vi "MTM2_issueCommand_setAuthList.vi"(8 "error in (no error)":errorcluster, 11 "command_setAuthList_Ctl":T1) -> (0 "error out":errorcluster, 2 "function return":i32, 3 "command_setAuthList_Ctl out":T1)   [LabVIEW 2018, in "SALLV_MTM2.lvlib"]
doc: "int MTM2_shm_issueCommand_setAuthListLV(MTM2_command_setAuthListLV *command_setAuthList_Ctl );"
uses:
  DataTypes/command_setAuthList.ctl
  SALLV_MTM2.lvlib
  SALLV_MTM2.so
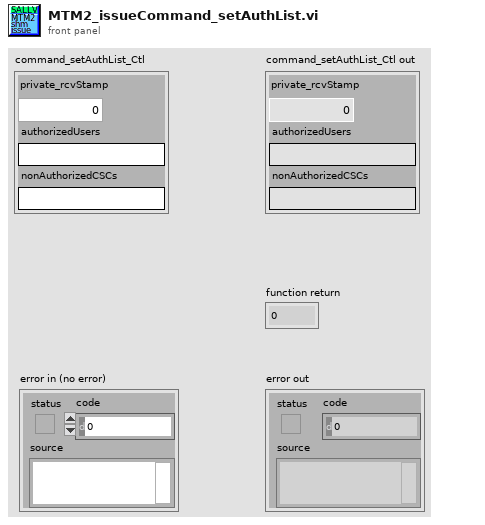
[diagram p1: front panel]
types:
  T1 = typedef "SALLV_MTM2.lvlib/command_setAuthList.ctl" = cluster{"private_rcvStamp":dbl, "authorizedUsers":string, "nonAuthorizedCSCs":string}
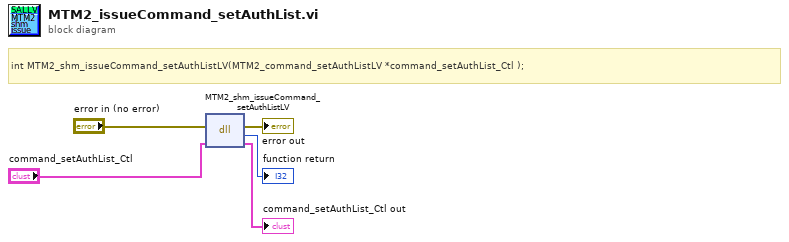
[diagram p0: block diagram]
diagram:
  # "int MTM2_shm_issueCommand_setAuthListLV(MTM2_command_setAuthListLV *command_setAuthList_Ctl );"
  n1 = dll-call lib="home/ttsai/Documents/salTestLabViewApi/SALLV_MTM2/SALLV_MTM2.*" fn="MTM2_shm_issueCommand_setAuthListLV"(error in="error in (no error)", "command_setAuthList_Ctl"="command_setAuthList_Ctl") -> (error out=→"error out":errorcluster, →"function return":i32, "command_setAuthList_Ctl"=→"command_setAuthList_Ctl out":T1)  [unwired: 2 in, 1 out]
